vi "ROI_Image_Create tangent line to circle.vi"(8 "error in (no error)":errorcluster, 9 "Orient rel to center":T2, 10 "Circles Data":T4, 11 "Intersection Point":cluster{"X":i32, "Y":i32}) -> (0 "error out":errorcluster, 1 "Line End Points":cluster{"X":dbl, "Y":dbl}[](array[cluster]), 2 "Tangent Line":T3 {"Point 2"."Y" format="%.2f"; "Point 2"."X" format="%.2f"; "Point 1"."Y" format="%.2f"; "Point 1"."X" format="%.2f"}, 4 "ROI":T1 {"Contours"."Type" items=["No Selection", "Point", "Line", "Rectangle", "Oval", "Polygon", "Freehand Region", "Annulus", "Unused2", "Unused3", "Broken Line", "Freehand Line", "Rotated Rectangle"]})   [LabVIEW 2012]
uses:
  custom controls/enum - StartPt Relative to Circle Center.ctl
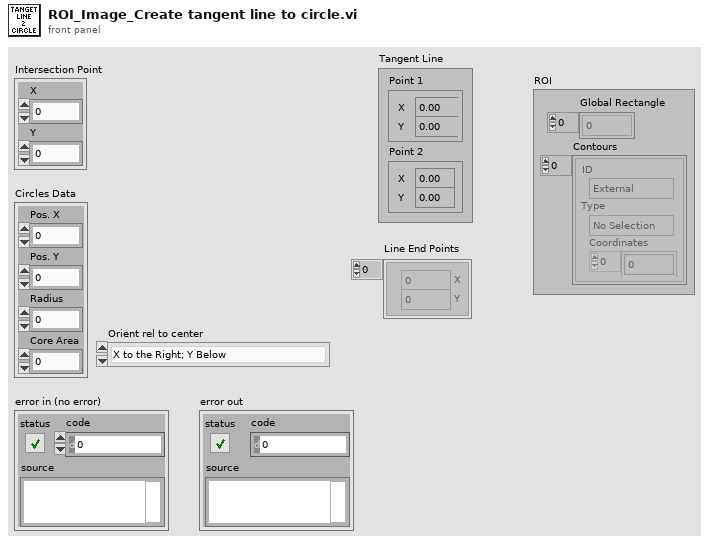
[diagram p1: front panel]
types:
  T1 = typedef "ROI Descriptor" = cluster{"Global Rectangle":i32[], "Contours":cluster{"ID":enum32{"External", "Internal"}, "Type":u32, "Coordinates":i32[]}[]}
  T2 = typedef "enum - StartPt Relative to Circle Center.ctl" = enum16{"X to the Right; Y Below", "X to the Right; Y Above", "X to the Left; Y Below", "X to the Left: Y Above"}
  T3 = cluster{"Point 1":cluster{"X":sgl, "Y":sgl}, "Point 2":cluster{"X":sgl, "Y":sgl}}
  T4 = cluster{"Pos. X":i32, "Pos. Y":i32, "Radius":i32, "Core Area":i32}
  T5 = cluster{"ID":enum32{"External", "Internal"}, "Type":u32, "Coordinates":i32[]}
  T6 = cluster{"ID":enum32{"External", "Internal"}, "Type":u32, "Coordinates":i32[]}[]
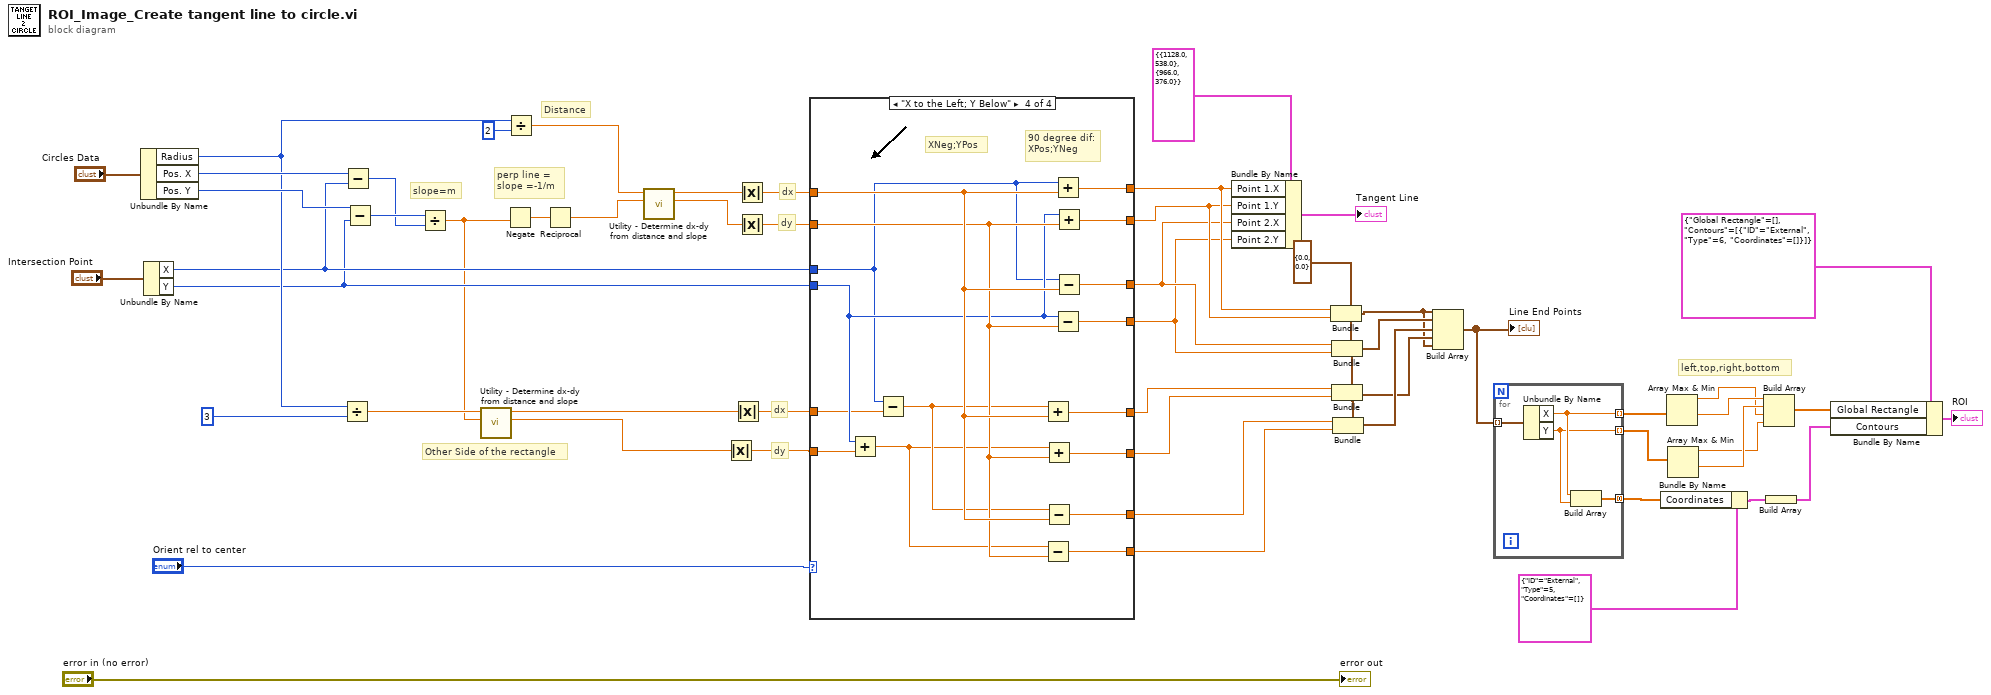
[diagram p0: block diagram]
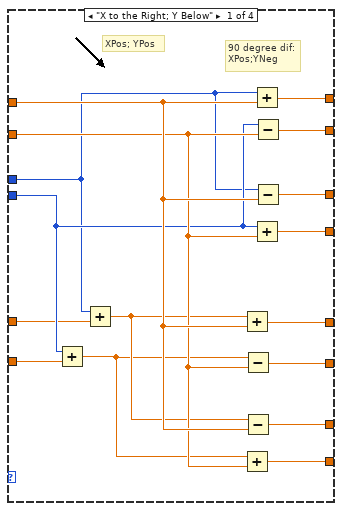
[diagram p2: hidden frame]
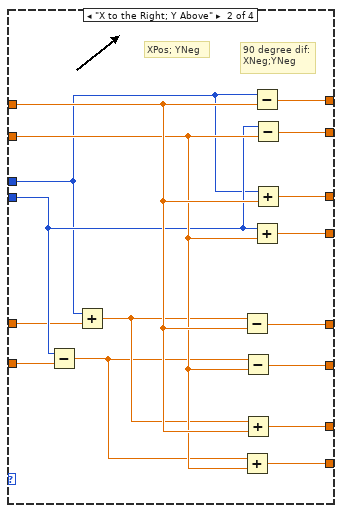
[diagram p3: hidden frame]
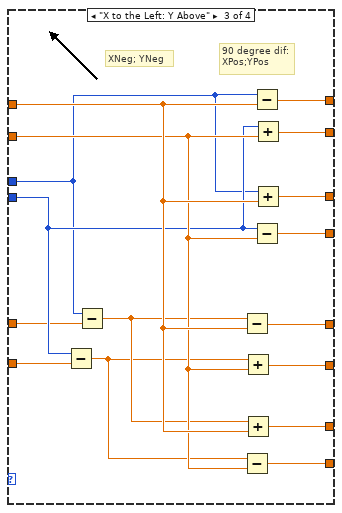
[diagram p4: hidden frame]
diagram:
  w16 = cluster{"X":dbl, "Y":dbl} {"X"=0.0, "Y"=0.0} ("Point Coordinates")
  # "left,top,right,bottom"
  # "Distance"
  # "dx"
  # "Other Side of the rectangle"
  # "dy"
  # "dy"
  # "dx"
  # "perp line =  \nslope =-1/m"
  # "slope=m"
  n1 = Unbundle By Name("Circles Data") -> ("Radius"=w42:i32, "Pos. X"=w52:i32, "Pos. Y"=w51:i32)
  n2 = Unbundle By Name("Intersection Point") -> ("X"=w41:i32, "Y"=w26:i32)
  n3 = Divide(x=w42, y=3) -> (x/y=w22:dbl)
  n4 = Subtract(x=w52, y=w41) -> (x-y=w49:i32)
  n5 = Subtract(x=w51, y=w26) -> (x-y=w50:i32)
  n6 = Divide(x=w50, y=w49) -> (x/y=w21:dbl)
  n7 = call "Utility - Determine dx-dy from distance and slope.vi"("Slope (dy/dx)"=w21, "Distance= r"=w22) -> ("dy"=w19:dbl, "dx"=w20:dbl)  [unwired: 8 in]
  n8 = Negate(x=w21) -> (-x=w48:dbl)
  n9 = Divide(x=w42, y=2) -> (x/y=w40:dbl)
  n10 = Reciprocal(x=w48) -> (1/x=w46:dbl)
  n11 = call "Utility - Determine dx-dy from distance and slope.vi"("Slope (dy/dx)"=w46, "Distance= r"=w40) -> ("dy"=w39:dbl, "dx"=w23:dbl)  [unwired: 8 in]
  n12 = Absolute Value(x=w19) -> (abs(x)=w18:dbl)
  n13 = Absolute Value(x=w20) -> (abs(x)=w25:dbl)
  n14 = Absolute Value(x=w23) -> (abs(x)=w17:dbl)
  n15 = Absolute Value(x=w39) -> (abs(x)=w24:dbl)
  n16 = case shown="\"X to the Left; Y Below\"" "Orient rel to center" {
    tunnel: w41 -> [w59 w75 w91 w107]
    tunnel: w26 -> [w60 w76 w92 w108]
    tunnel: w17 -> [w71 w87 w103 w119]
    tunnel: w24 -> [w70 w86 w102 w118]
    tunnel: [w69 w85 w101 w117] -> w38
    tunnel: [w68 w84 w100 w116] -> w37
    tunnel: [w67 w83 w99 w115] -> w36
    tunnel: [w66 w82 w98 w114] -> w35
    tunnel: [w65 w81 w97 w113] -> w33
    tunnel: [w64 w80 w96 w112] -> w32
    tunnel: [w63 w79 w95 w111] -> w31
    tunnel: [w62 w78 w94 w110] -> w30
    tunnel: w18 -> [w61 w77 w93 w109]
    tunnel: w25 -> [w58 w74 w90 w106]
    frame "X to the Right; Y Below" {
      # "90 degree dif:\nXPos;YNeg"
      # "XPos; YPos"
      n17 = Add(x=w60, y=w61) -> (x+y=w56:dbl)
      n18 = Add(x=w59, y=w58) -> (x+y=w57:dbl)
      n19 = Add(x=w57, y=w71) -> (x+y=w65:dbl)
      n20 = Add(x=w56, y=w70) -> (x+y=w62:dbl)
      n21 = Subtract(x=w56, y=w70) -> (x-y=w64:dbl)
      n22 = Subtract(x=w57, y=w71) -> (x-y=w63:dbl)
      n23 = Add(x=w59, y=w71) -> (x+y=w69:dbl)
      n24 = Add(x=w60, y=w70) -> (x+y=w66:dbl)
      n25 = Subtract(x=w60, y=w70) -> (x-y=w68:dbl)
      n26 = Subtract(x=w59, y=w71) -> (x-y=w67:dbl)
    }
    frame "X to the Right; Y Above" {
      # "90 degree dif:\nXNeg;YNeg"
      # "XPos; YNeg"
      n27 = Subtract(x=w76, y=w77) -> (x-y=w72:dbl)
      n28 = Add(x=w75, y=w74) -> (x+y=w73:dbl)
      n29 = Subtract(x=w73, y=w87) -> (x-y=w81:dbl)
      n30 = Add(x=w72, y=w86) -> (x+y=w78:dbl)
      n31 = Subtract(x=w72, y=w86) -> (x-y=w80:dbl)
      n32 = Add(x=w73, y=w87) -> (x+y=w79:dbl)
      n33 = Subtract(x=w75, y=w87) -> (x-y=w85:dbl)
      n34 = Add(x=w76, y=w86) -> (x+y=w82:dbl)
      n35 = Subtract(x=w76, y=w86) -> (x-y=w84:dbl)
      n36 = Add(x=w75, y=w87) -> (x+y=w83:dbl)
    }
    frame "X to the Left: Y Above" {
      # "90 degree dif:\nXPos;YPos"
      # "XNeg; YNeg"
      n37 = Subtract(x=w92, y=w93) -> (x-y=w88:dbl)
      n38 = Subtract(x=w91, y=w90) -> (x-y=w89:dbl)
      n39 = Subtract(x=w89, y=w103) -> (x-y=w97:dbl)
      n40 = Subtract(x=w88, y=w102) -> (x-y=w94:dbl)
      n41 = Add(x=w88, y=w102) -> (x+y=w96:dbl)
      n42 = Add(x=w89, y=w103) -> (x+y=w95:dbl)
      n43 = Subtract(x=w91, y=w103) -> (x-y=w101:dbl)
      n44 = Subtract(x=w92, y=w102) -> (x-y=w98:dbl)
      n45 = Add(x=w92, y=w102) -> (x+y=w100:dbl)
      n46 = Add(x=w91, y=w103) -> (x+y=w99:dbl)
    }
    frame "X to the Left; Y Below" {
      # "90 degree dif:\nXPos;YNeg"
      # "XNeg;YPos"
      n47 = Add(x=w108, y=w109) -> (x+y=w104:dbl)
      n48 = Subtract(x=w107, y=w106) -> (x-y=w105:dbl)
      n49 = Add(x=w105, y=w119) -> (x+y=w113:dbl)
      n50 = Subtract(x=w104, y=w118) -> (x-y=w110:dbl)
      n51 = Add(x=w104, y=w118) -> (x+y=w112:dbl)
      n52 = Subtract(x=w105, y=w119) -> (x-y=w111:dbl)
      n53 = Add(x=w107, y=w119) -> (x+y=w117:dbl)
      n54 = Subtract(x=w108, y=w118) -> (x-y=w114:dbl)
      n55 = Add(x=w108, y=w118) -> (x+y=w116:dbl)
      n56 = Subtract(x=w107, y=w119) -> (x-y=w115:dbl)
    }
  }
  n57 = Bundle By Name(cluster=T3 {"Point 1"={"X"=1128.0, "Y"=538.0}, "Point 2"={"X"=966.0, "Y"=376.0}} ("Tangent Line"), "Point 1.X"=w38, "Point 1.Y"=w37, "Point 2.X"=w36, "Point 2.Y"=w35) -> (→"Tangent Line":T3)
  n58 = Bundle(cluster=w16, "X"=w38, "Y"=w37) -> (w2:cluster{"X":dbl, "Y":dbl})
  n59 = Bundle(cluster=w16, "X"=w36, "Y"=w35) -> (w34:cluster{"X":dbl, "Y":dbl})
  n60 = Bundle(cluster=w16, "X"=w33, "Y"=w32) -> (w28:cluster{"X":dbl, "Y":dbl})
  n61 = Bundle(cluster=w16, "X"=w31, "Y"=w30) -> (w29:cluster{"X":dbl, "Y":dbl})
  n62 = Build Array(w2, w34, w29, w28, w2) -> (w1:cluster{"X":dbl, "Y":dbl}[])
  "Line End Points" <- w1
  n63 = for {
    tunnel: w1 -> [w123] mode=indexing
    tunnel: [w122] -> w15 mode=indexing
    tunnel: [w121] -> w14 mode=indexing
    tunnel: [w120] -> w6 mode=concatenating
    n64 = Unbundle By Name(w123) -> ("X"=w122:dbl, "Y"=w121:dbl)
    n65 = Build Array(w122, w121) -> (w120:dbl[])
  }
  n66 = Bundle By Name(cluster=T5 {"ID"=enum."External", "Type"=5, "Coordinates"=[]}, "Coordinates"=w6) -> (w5:T5)
  n67 = Array Max & Min(array=w15) -> (max value=w11:dbl, min value=w13:dbl)  [unwired: 2 out]
  n68 = Array Max & Min(array=w14) -> (max value=w10:dbl, min value=w12:dbl)  [unwired: 2 out]
  n69 = Build Array(w13, w12, w11, w10) -> (w8:dbl[])
  n70 = Build Array(w5) -> (w4:T6)
  n71 = Bundle By Name(cluster=T1 {"Global Rectangle"=[], "Contours"=[{"ID"=enum."External", "Type"=6, "Coordinates"=[]}]} ("ROI Descriptor"), "Global Rectangle"=w8, "Contours"=w4) -> (→"ROI":T1)
  "error out" <- "error in (no error)"
